vi "Initialise Thrust Dots.vi"(11 "Ship in":refnum<class "Ship.lvclass">) -> (3 "Ship out":refnum<class "Ship.lvclass">)   [LabVIEW 2021, in "Ship.lvclass"]
uses:
  Ship.lvclass
  Ship.lvclass/Ship.ctl
  Thrust Dot/Thrust Dot.lvclass
  Vector 2D/Vector 2D.lvclass
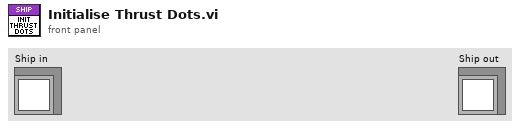
[diagram p1: front panel]
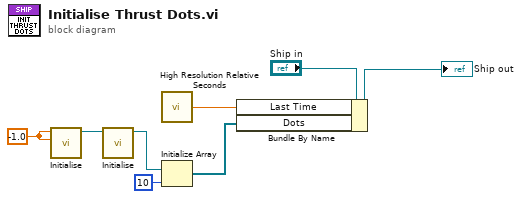
[diagram p0: block diagram]
diagram:
  w1 = sgl -1.0 ("x")
  n1 = call "Initialise.vi"("y"=w1, "x"=w1) -> ("Vector 2D out"=w2:refnum<class "Vector 2D.lvclass">)  [unwired: 9 in]
  n2 = call "Initialise.vi"("Position"=w2) -> ("Thrust Dot out"=w3:refnum<class "Thrust Dot.lvclass">)  [unwired: 10 in]
  n3 = call <vilib>:"High Resolution Relative Seconds.vi"() -> ("relative seconds"=w6:dbl)
  n4 = Initialize Array(w3, 10 ("dimension size")) -> (w4:refnum<class "Thrust Dot.lvclass">[])
  n5 = Bundle By Name(cluster="Ship in", "Last Time"=w6, "Dots"=w4) -> (→"Ship out":refnum<class "Ship.lvclass">)
